vi "PID_position (SubVI).vi"(9 "PID gains in":T1={"proportional gain (Kc)"=1.0, "integral time (Ti, min)"=0.01, "derivative time (Td, min)"=0.0} {"derivative time (Td, min)" format="%.3f"; "integral time (Ti, min)" format="%.3f"; "proportional gain (Kc)" format="%.3f"}, 10 "setpoint":dbl format="%.2f", 11 "Voltage Range in":cluster{"output high":dbl, "output low":dbl}={"output high"=100.0, "output low"=-100.0} {"output low" format="%.2f"; "output high" format="%.2f"}) -> (3 "Vout":dbl format="%.2f")   [LabVIEW 2015]
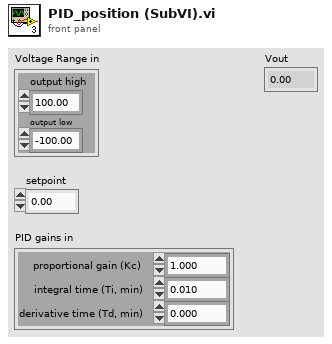
[diagram p1: front panel]
types:
  T1 = cluster{"proportional gain (Kc)":dbl, "integral time (Ti, min)":dbl, "derivative time (Td, min)":dbl}
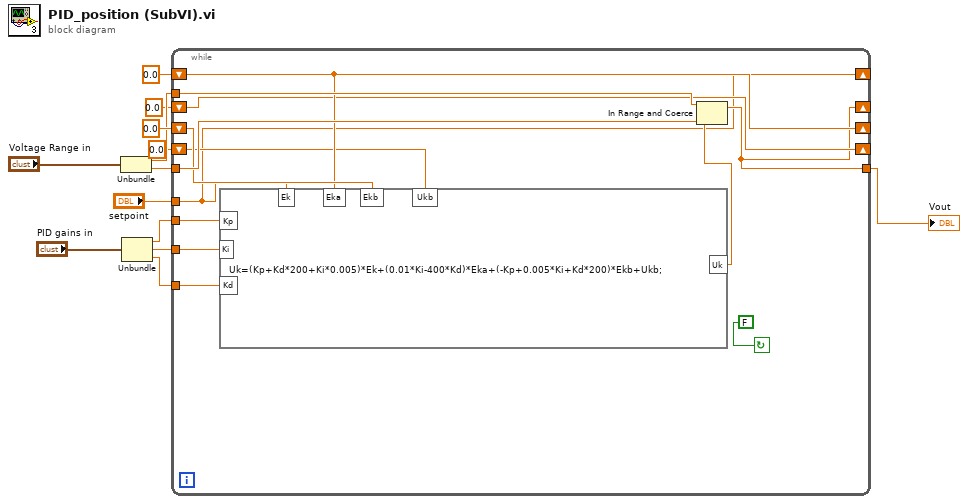
[diagram p0: block diagram]
diagram:
  n1 = Unbundle("Voltage Range in") -> ("output high"=w6:dbl, "output low"=w7:dbl)
  n2 = Unbundle("PID gains in") -> ("proportional gain (Kc)"=w3:dbl, "integral time (Ti, min)"=w4:dbl, "derivative time (Td, min)"=w5:dbl)
  n3 = while {
    shift-right: [w14] -> _
    shift-left: 0.0 -> [w19]
    tunnel: w3 -> [w25]
    tunnel: w4 -> [w24]
    tunnel: w5 -> [w23]
    tunnel: w6 -> [w21]
    tunnel: w7 -> [w22]
    tunnel: "setpoint" -> [w14]
    tunnel: [w15] -> w12
    shift-right: [w19] -> _
    shift-left: 0.0 -> [w20]
    shift-right: [w15] -> _
    shift-left: 0.0 ("output high") -> [w17]
    shift-right: [w17] -> _
    shift-left: 0.0 ("output high") -> [w16]
    stop <- FALSE continue-if-true
    n4 = formula code="Uk=(Kp+Kd*200+Ki*0.005)*Ek+(0.01*Ki-400*Kd)*Eka+(-Kp+0.005*Ki+Kd*200)*Ekb+Ukb;"("Kp"=w25, "Ki"=w24, "Kd"=w23, "Ek"=w14, "Eka"=w19, "Ekb"=w20, "Ukb"=w16) -> ("Uk"=w18:dbl)
    n5 = In Range and Coerce(upper limit=w21, x=w18, lower limit=w22) -> (coerced(x)=w15:dbl)  [unwired: 1 out]
  }
  "Vout" <- w12
